vi "Find QWTB Error.vi"(8 "error in (no error)":errorcluster) -> (0 "error out":errorcluster, 2 "Internal QWTB error":bool, 3 "QWTB error\n(empty string)":string)   [LabVIEW 2013, in "QWTBLVLib.lvlib"]
doc: "Checks if error in contains QWTB error. If so, parse it and produce a string containing only QWTB error."
uses:
  QWTBLVLib.lvlib
  <vilib>/regexp/Match Regular Expression.xnode
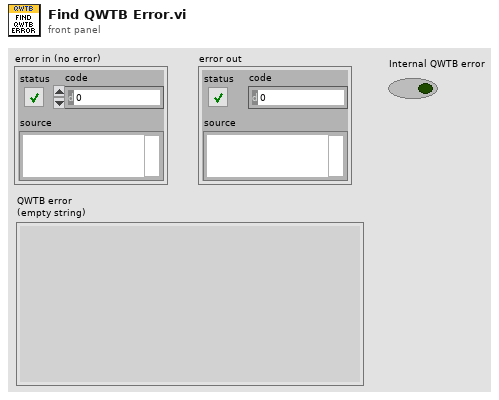
[diagram p1: front panel]
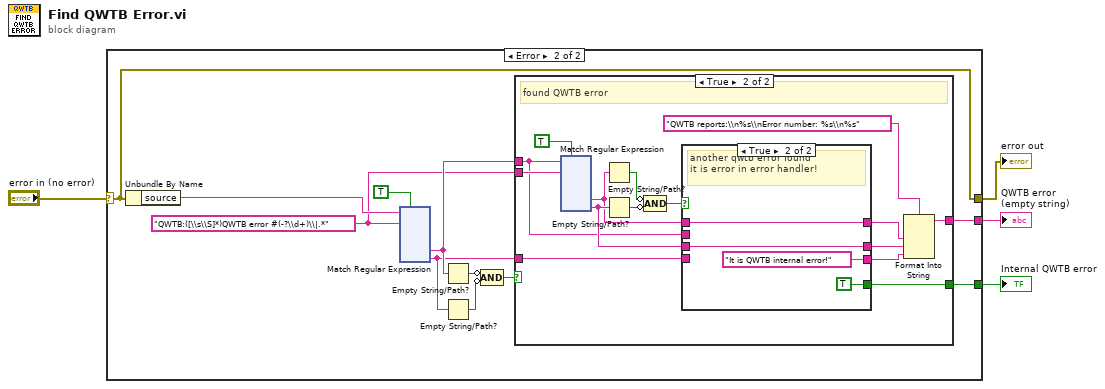
[diagram p0: block diagram]
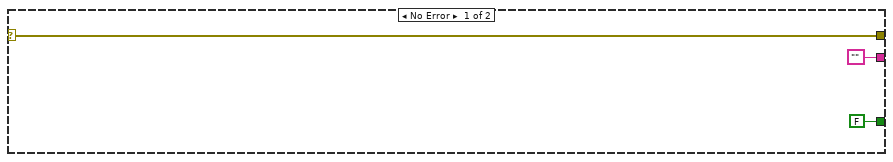
[diagram p2: hidden frame]
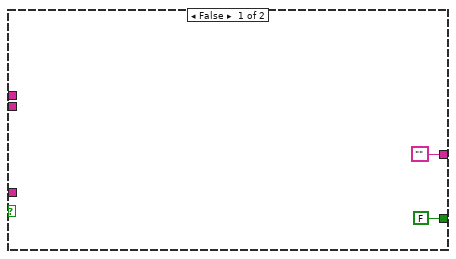
[diagram p3: hidden frame]
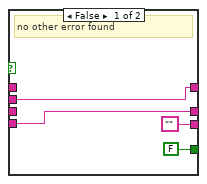
[diagram p4: hidden frame]
diagram:
  n1 = case shown="Error" "error in (no error)" {
    selector: "error in (no error)" -> [w7 w9]
    tunnel: [w7 w9] -> w4
    tunnel: ["" w10] -> w2
    tunnel: [FALSE ("Internal QWTB error") w8] -> w1
    frame No Error {
    }
    frame Error {
      w13 = "QWTB:([\\s\\S]*)QWTB error #(-?\\d+)\\|.*" ("regular expression")
      n2 = Unbundle By Name(w9) -> ("source"=w18:string)
      n3 = xnode "Match Regular Expression"("input string"=w18, "regular expression"=w13, "ignore case? (F)"=TRUE) -> ("submatch 1"=w14:string, "submatch 2"=w11:string)  [unwired: 3 in, 5 out]
      n4 = Empty String/Path?(string/path=w14) -> (empty?=w17:bool)
      n5 = Empty String/Path?(string/path=w11) -> (empty?=w16:bool)
      n6 = Compound Arithmetic op=AND(invert w17, invert w16) -> (w15:bool)
      n7 = case shown="True" w15 {
        tunnel: w14 -> [_ w28]
        tunnel: w13 -> [_ w35]
        tunnel: w11 -> [_ w27]
        tunnel: ["" w22] -> w10
        tunnel: [FALSE ("Internal QWTB error") w21] -> w8
        frame False {
        }
        frame True {
          # "found QWTB error"
          n8 = xnode "Match Regular Expression"("input string"=w28, "regular expression"=w35, "ignore case? (F)"=TRUE) -> ("submatch 1"=w29:string, "submatch 2"=w30:string)  [unwired: 3 in, 5 out]
          n9 = Empty String/Path?(string/path=w29) -> (empty?=w33:bool)
          n10 = Empty String/Path?(string/path=w30) -> (empty?=w34:bool)
          n11 = Compound Arithmetic op=AND(invert w33, invert w34) -> (w31:bool)
          n12 = case shown="True" w31 {
            tunnel: w30 -> [_ w43]
            tunnel: w29 -> [_ w42]
            tunnel: w28 -> [w39 _]
            tunnel: w27 -> [w38 _]
            tunnel: [w38 w43] -> w24
            tunnel: [w39 w42] -> w25
            tunnel: ["" "It is QWTB internal error!" ("format string")] -> w23
            tunnel: [FALSE ("Internal QWTB error") TRUE ("Internal QWTB error")] -> w21
            frame False {
              # "no other error found"
            }
            frame True {
              # "another qwtb error found\nit is error in error handler!"
            }
          }
          n13 = Format Into String(format string="QWTB reports:\\n%s\\nError number: %s\\n%s", w25, w24, w23) -> (resulting string=w22:string)  [unwired: 2 in, 1 out]
        }
      }
    }
  }
  "error out" <- w4
  "QWTB error\n(empty string)" <- w2
  "Internal QWTB error" <- w1
